vi "SeCrTS-DD NS Data Storage.vi"(7 "NOT DIS Out":T1, 8 "value 2":T2, 9 "AI_V_Data P\nAI_C_Data P\nAO_Data P\nDO_Data P\nACC_Data P\nTC Data P\nDrive_A_C \nDrive_A_D\nAI_C_Data S\nDO_Data S":refnum<queue>[](array[refnum]), 11 "DI P\nDI S":refnum<queue>[](array[refnum])) -> ()   [LabVIEW 2022 SP3]
uses:
  Control/SeCrTS-Notifier Ref.ctl
panel:
  out "overflow? 5":bool
  out "overflow? 3":bool
  out "overflow? 2":bool
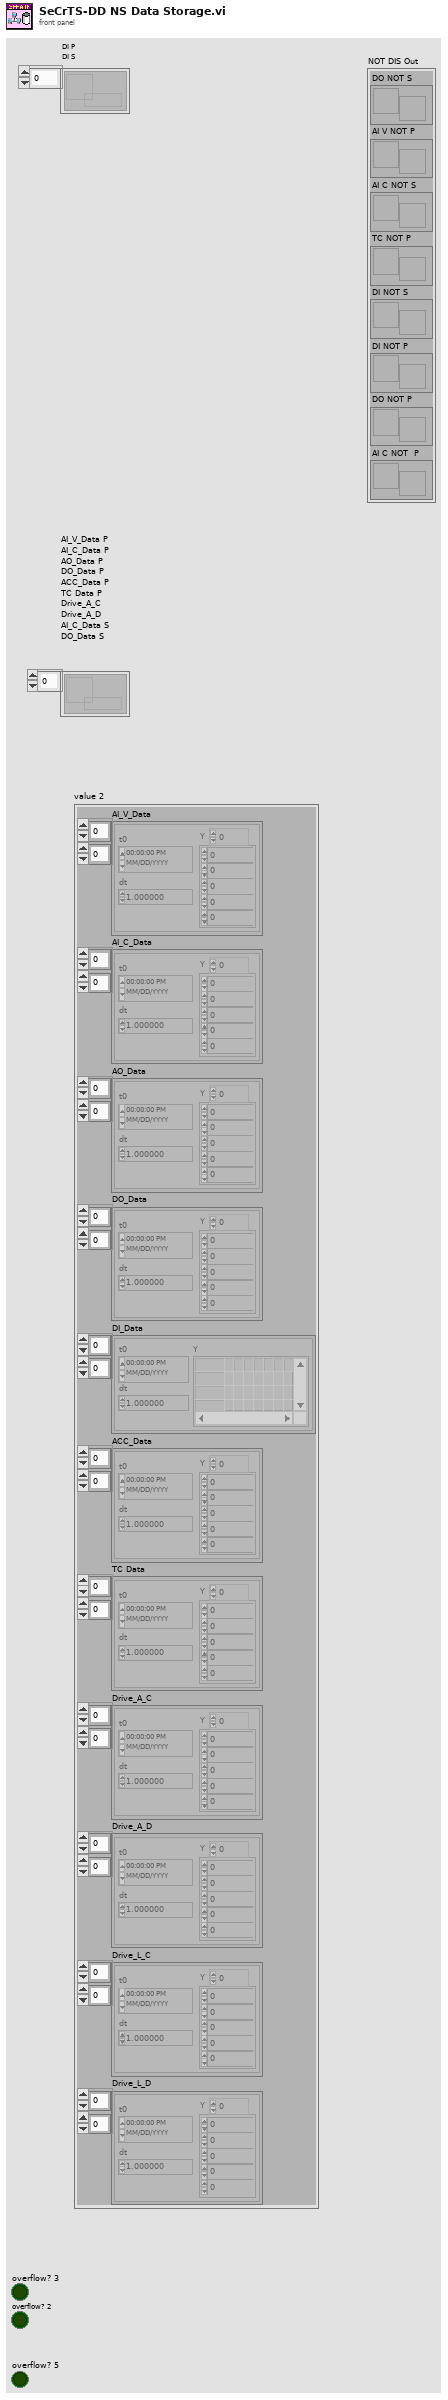
[diagram p1: front panel]
types:
  T1 = typedef "SeCrTS-Notifier Ref.ctl" = cluster{"DO NOT S":refnum<notifier>, "AI V NOT P":refnum<notifier>, "AI C NOT S":refnum<notifier>, "TC NOT P":refnum<notifier>, "DI NOT S":refnum<notifier>, "DI NOT P":refnum<notifier>, "DO NOT P":refnum<notifier>, "AI C NOT  P":refnum<notifier>}
  T2 = cluster{"AI_V_Data":waveform(dbl)[][], "AI_C_Data":waveform(dbl)[][], "AO_Data":waveform(dbl)[][], "DO_Data":waveform(dbl)[][], "DI_Data":digitalwaveform[][], "ACC_Data":waveform(dbl)[][], "TC Data":waveform(dbl)[][], "Drive_A_C":waveform(dbl)[][], "Drive_A_D":waveform(dbl)[][], "Drive_L_C":waveform(dbl)[][], "Drive_L_D":waveform(dbl)[][]}
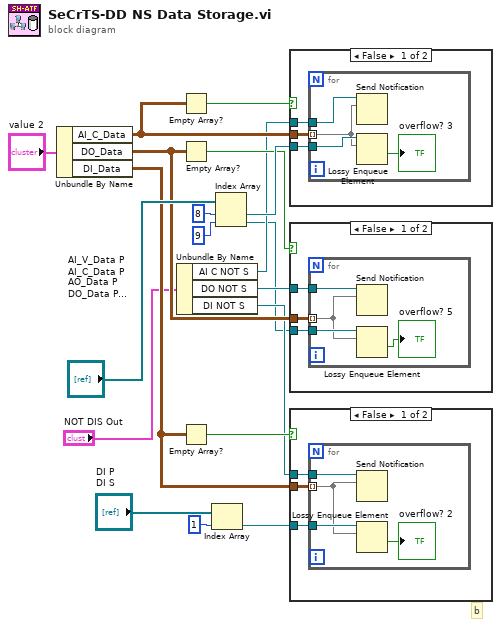
[diagram p0: block diagram]
diagram:
  # "b"
  n1 = Unbundle By Name("value 2") -> ("AI_C_Data"=w13:waveform(dbl)[][], "DO_Data"=w10:waveform(dbl)[][], "DI_Data"=w15:digitalwaveform[][])
  n2 = Unbundle By Name("NOT DIS Out") -> ("AI C NOT S"=w9:refnum<notifier>, "DO NOT S"=w8:refnum<notifier>, "DI NOT S"=w7:refnum<notifier>)
  n3 = Empty Array?(array=w13) -> (empty?=w14:bool)
  n4 = Empty Array?(array=w10) -> (empty?=w11:bool)
  n5 = Empty Array?(array=w15) -> (empty?=w16:bool)
  n6 = Index Array(array="DI P\nDI S", index=1) -> (element=w2:refnum<queue>)
  n7 = Index Array(array="AI_V_Data P\nAI_C_Data P\nAO_Data P\nDO_Data P\nACC_Data P\nTC Data P\nDrive_A_C \nDrive_A_D\nAI_C_Data S\nDO_Data S", index #1=8 ("index"), index #2=9 ("index")) -> (element #1=w18:refnum<queue>, element #2=w4:refnum<queue>)
  n8 = case shown="False" w14 {
    tunnel: w13 -> [w22 _]
    tunnel: w18 -> [w21 _]
    tunnel: w9 -> [w20 _]
    frame False {
      n9 = for {
        tunnel: w22 -> [w23] mode=indexing
        tunnel: w21 -> [w26]
        tunnel: w20 -> [w24]
        n10 = Send Notification(notification=w23, notifier=w24) -> ()  [unwired: 1 in, 2 out]
        n11 = Lossy Enqueue Element(queue=w26, element=w23) -> (overflow?=→"overflow? 3":bool)  [unwired: 1 in, 3 out]
      }
    }
    frame True {
    }
  }
  n12 = case shown="False" w11 {
    tunnel: w10 -> [w29 _]
    tunnel: w4 -> [w28 _]
    tunnel: w8 -> [w27 _]
    frame False {
      n13 = for {
        tunnel: w29 -> [w30] mode=indexing
        tunnel: w28 -> [w33]
        tunnel: w27 -> [w31]
        n14 = Send Notification(notification=w30, notifier=w31) -> ()  [unwired: 1 in, 2 out]
        n15 = Lossy Enqueue Element(queue=w33, element=w30) -> (overflow?=→"overflow? 5":bool)  [unwired: 1 in, 3 out]
      }
    }
    frame True {
    }
  }
  n16 = case shown="False" w16 {
    tunnel: w15 -> [w36 _]
    tunnel: w2 -> [w35 _]
    tunnel: w7 -> [w34 _]
    frame False {
      n17 = for {
        tunnel: w36 -> [w37] mode=indexing
        tunnel: w35 -> [w40]
        tunnel: w34 -> [w38]
        n18 = Send Notification(notification=w37, notifier=w38) -> ()  [unwired: 1 in, 2 out]
        n19 = Lossy Enqueue Element(queue=w40, element=w37) -> (overflow?=→"overflow? 2":bool)  [unwired: 1 in, 3 out]
      }
    }
    frame True {
    }
  }
